vi "Read Remaining Samples.vi"(8 "error in (no error)":errorcluster, 11 "SV Signal in":refnum<class "SV Signal.lvclass">) -> (0 "error out":errorcluster, 2 "remaining samples":i32, 3 "SV Signal out":refnum<class "SV Signal.lvclass">)   [LabVIEW 2017, in "SV Signal.lvclass"]
uses:
  <vilib>/addons/_NISVFA/_Generation/Signal Generation/SV Signal/SV Signal.lvclass
  <vilib>/addons/_NISVFA/_Generation/Signal Generation/SV Signal/SV Signal.lvclass/SV Signal.ctl
  <vilib>/addons/_NISVFA/_Generation/Signal Generation/SV Signal/Read System Timing Model.vi
  <vilib>/addons/_NISVFA/_Generation/Signal Generation/SV Signal/Read Generation State.vi
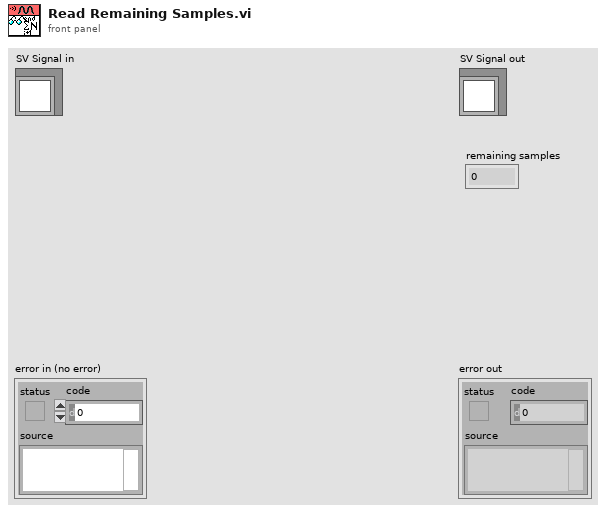
[diagram p1: front panel]
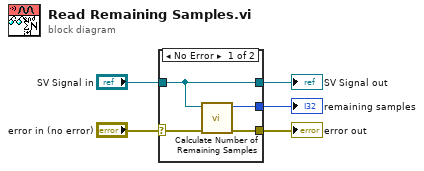
[diagram p0: block diagram]
diagram:
  n1 = case shown="No Error" "error in (no error)" {
    selector: "error in (no error)" -> [w9 w11]
    tunnel: [w8 w11] -> w4
    tunnel: [w6 w10] -> w2
    tunnel: "SV Signal in" -> [w6 w10]
    tunnel: [w7 _] -> w1
    frame No Error {
      n2 = call <vilib>:"Calculate Number of Remaining Samples.vi"("error in (no error)"=w9, "SV Signal in"=w6) -> ("error out"=w8:errorcluster, "remaining samples"=w7:i32)  [unwired: 8 in]
    }
    frame Error {
    }
  }
  "error out" <- w4
  "SV Signal out" <- w2
  "remaining samples" <- w1
